vi "SeCrTs-DO_Scale.vi"(8 "error in (no error)":errorcluster, 10 "DO":T1(array[cluster]), 11 "Refnum in":refnum<k21>) -> (0 "error out":errorcluster, 2 "Array":bool[](array[boolean]), 3 "Refnum out":refnum<k21>)   [LabVIEW 2022 SP3]
uses:
  <vilib>/DAQmx/create/channels.llb/DAQmx Create Channel (DO-Digital Output).vi
  <resource>/objmgr/daqmx.rc
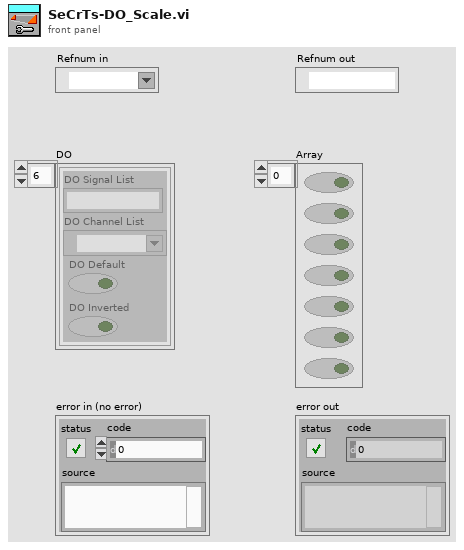
[diagram p1: front panel]
types:
  T1 = cluster{"DO Signal List":string, "DO Channel List":tag, "DO Default":bool, "DO Inverted":bool}[]
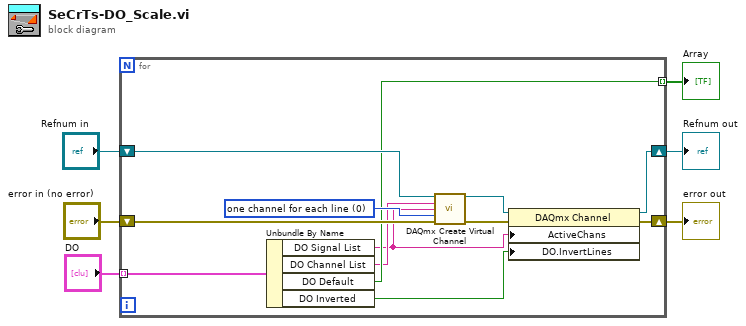
[diagram p0: block diagram]
diagram:
  n1 = for {
    tunnel: "DO" -> [w18] mode=indexing
    shift-right: [w12] -> w1
    shift-left: "Refnum in" -> [w17]
    shift-right: [w11] -> w2
    shift-left: "error in (no error)" -> [w16]
    tunnel: [w14] -> w3 mode=indexing
    w15 = 0 items=["one channel for each line", "one channel for all lines"] ("line grouping")
    n2 = Unbundle By Name(w18) -> ("DO Signal List"=w8:string, "DO Channel List"=w9:tag, "DO Default"=w14:bool, "DO Inverted"=w7:bool)
    n3 = call-poly <vilib>:"DAQmx Create Virtual Channel.vi"("task in"=w17, "lines"=w9, "name to assign"=w8, "line grouping"=w15, "error in"=w16) -> ("task out"=w13:refnum<k21>, "error out"=w10:errorcluster)  [unwired: 9 in]
    n4 = property on="Property Node" class="DAQmx Channel"(reference=w13, error in=w10, "ActiveChans"=w8, "DO.InvertLines"=w7) -> (reference out=w12:refnum<k21>, error out=w11:errorcluster)
  }
  "Array" <- w3
  "error out" <- w2
  "Refnum out" <- w1
